vi "MGI U8 Data to Hex Str.vi"(1 "u8 Data[]":u8[](array[numeric]) format="%.0x") -> (0 "HEX String (0-9,A-F)":string)   [LabVIEW 2020, in "PixPack.lvlib"]
doc: "Convert the array of bytes to a Hex String containing 0-9 and A-F. This VI is optimized for large input arrays.\n\nAuthored by Shawn Walpole\nsupport@mooregoodideas.com\nwww.mooregoodideas.com\n\nCopyright (c) 2010, Moore Good Ideas, Inc.\n\nAll rights reserved.\n\nRedistribution and use in source and binary forms, with or without modification, are permitted provided that the following conditions are met:\n\n * Redistributions of source code must retain the above copyright notice, this list of conditions and the following disclaimer.\n * Redistributions in binary form must reproduce the above copyright notice, this list of conditions and the following disclaimer in the documentation and/or other materials provided with the distribution.\n * Neither the name of Moore Good Ideas, Inc. nor the names of its contributors may be used to endorse or promote products derived from this software without specific prior written permission.\n\nTHIS SOFTWARE IS PROVIDED BY THE COPYRIGHT HOLDERS AND CONTRIBUTORS \"AS IS\" AND ANY EXPRESS OR IMPLIED WARRANTIES, INCLUDING, BUT NOT LIMITED TO, THE IMPLIED WARRANTIES OF MERCHANTABILITY AND FITNESS FOR A PARTICULAR PURPOSE ARE DISCLAIMED. IN NO EVENT SHALL THE COPYRIGHT OWNER OR CONTRIBUTORS BE LIABLE FOR ANY DIRECT, INDIRECT, INCIDENTAL, SPECIAL, EXEMPLARY, OR CONSEQUENTIAL DAMAGES (INCLUDING, BUT NOT LIMITED TO, PROCUREMENT OF SUBSTITUTE GOODS OR SERVICES; LOSS OF USE, DATA, OR PROFITS; OR BUSINESS INTERRUPTION) HOWEVER CAUSED AND ON ANY THEORY OF LIABILITY, WHETHER IN CONTRACT, STRICT LIABILITY, OR TORT (INCLUDING NEGLIGENCE OR OTHERWISE) ARISING IN ANY WAY OUT OF THE USE OF THIS SOFTWARE, EVEN IF ADVISED OF THE POSSIBILITY OF SUCH DAMAGE."
uses:
  PixPack.lvlib
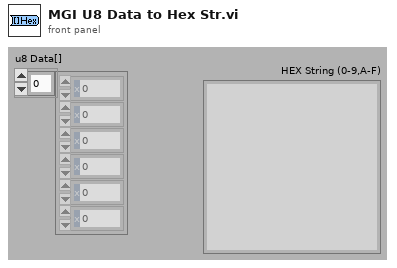
[diagram p1: front panel]
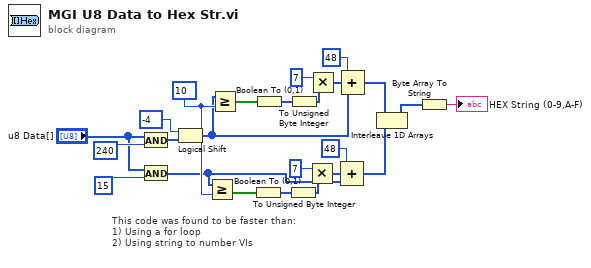
[diagram p0: block diagram]
diagram:
  w20 = u8 10
  # "This code was found to be faster than:\n1) Using a for loop\n2) Using string to number VIs"
  n1 = And(x="u8 Data[]", y=u8 240) -> (x .and. y?=w22:u8[])
  n2 = And(x="u8 Data[]", y=u8 15) -> (x .and. y?=w4:u8[])
  n3 = Logical Shift(y=i8 -4, x=w22) -> (x << y=w13:u8[])
  n4 = Greater Or Equal?(x=w4, y=w20) -> (x >= y?=w5:bool[])
  n5 = Greater Or Equal?(x=w13, y=w20) -> (x >= y?=w14:bool[])
  n6 = Boolean To (0,1)(Boolean=w5) -> (0, 1=w7:i16[])
  n7 = Boolean To (0,1)(Boolean=w14) -> (0, 1=w19:i16[])
  n8 = To Unsigned Byte Integer(number=w7) -> (unsigned 8bit integer=w8:u8[])
  n9 = To Unsigned Byte Integer(number=w19) -> (unsigned 8bit integer=w18:u8[])
  n10 = Multiply(x=u8 7, y=w8) -> (x*y=w10:u8[])
  n11 = Multiply(x=u8 7, y=w18) -> (x*y=w16:u8[])
  n12 = Compound Arithmetic op=ADD(u8 48, w10, w4) -> (w3:u8[])
  n13 = Compound Arithmetic op=ADD(u8 48, w16, w13) -> (w12:u8[])
  n14 = Interleave 1D Arrays(w12, w3) -> (w11:u8[])
  n15 = Byte Array To String(unsigned byte array=w11) -> (string=→"HEX String (0-9,A-F)":string)
